vi "Read Graph History.vi"(8 "error in (no error)":errorcluster, 11 "MFC in":refnum<class "MFC.lvclass">) -> (0 "error out":errorcluster, 2 "Graph History":refnum<vi>, 3 "MFC out":refnum<class "MFC.lvclass">)   [LabVIEW 2013, in "MFC.LVLIB" / "MFC.lvclass"]
uses:
  MFC.lvclass
  MFC.lvclass/MFC.ctl
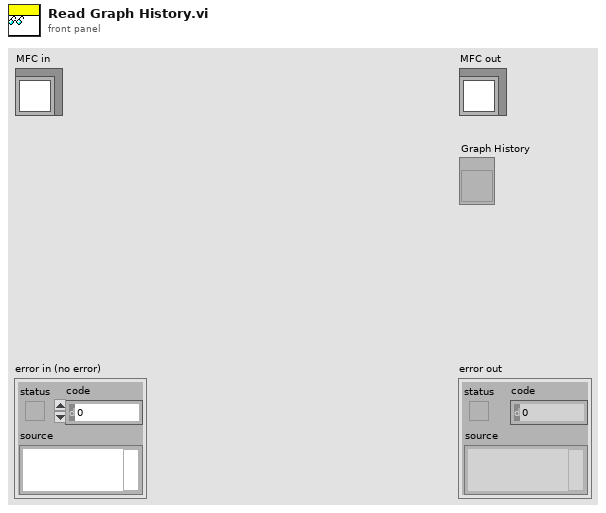
[diagram p1: front panel]
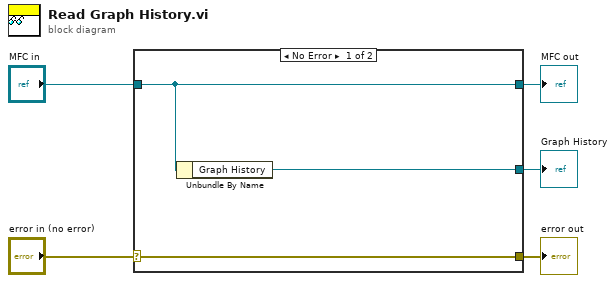
[diagram p0: block diagram]
diagram:
  n1 = case shown="No Error" "error in (no error)" {
    selector: "error in (no error)" -> [w8 w9]
    tunnel: [w8 w9] -> w4
    tunnel: [w7 w10] -> w2
    tunnel: "MFC in" -> [w7 w10]
    tunnel: [w6 _] -> w1
    frame No Error {
      n2 = Unbundle By Name(w7) -> ("Graph History"=w6:refnum<vi>)
    }
    frame Error {
    }
  }
  "error out" <- w4
  "MFC out" <- w2
  "Graph History" <- w1
